vi "<td>Array.vi"(11 "tableIn":string) -> (2 "remainingTable":string, 3 "firstRow":string[](array[string]))   [LabVIEW 2016]
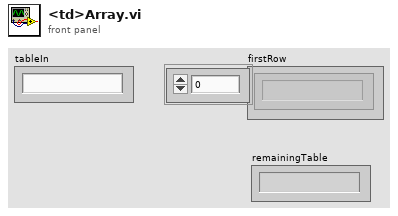
[diagram p1: front panel]
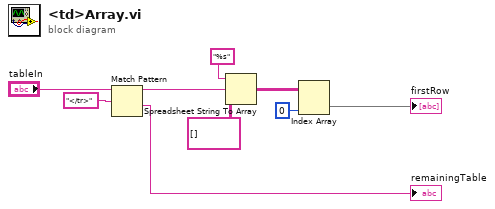
[diagram p0: block diagram]
diagram:
  n1 = Match Pattern(string="tableIn", regular expression="</tr>") -> (before substring=w4:string, after substring=→"remainingTable":string)  [unwired: 3 out]
  n2 = Spreadsheet String To Array(format string="%s", spreadsheet string=w4, array type (2D Dbl)=string[][] []) -> (array=w7:string[][])  [unwired: 1 in]
  n3 = Index Array(array=w7, index (col)=0 ("disabled index (col)")) -> (element=→"firstRow":string[])  [unwired: 1 in]
